vi "UI Main.vi"() -> ()   [LabVIEW 2020]
uses:
  controls/Control Configuration.ctl
  controls/UI Data.ctl
  controls/All FPGA Configuration Values.ctl
  controls/FPGA State.ctl
  controls/Raw Values.ctl
  Globals/Global - All UI Loop Stop.vi
  Globals/Global - UI Stream and Variable Connections.vi
  Globals/Global - Configuration Options.vi
  support/User Event - Stop/User Event - Stop.lvlib
  support/Message Queue/Message Queue.lvlib
panel:
  in  "Switch to Safe State":bool
  in  "Exit":bool
  out "System Status":string
  out "Current FPGA Control Mode":u16(ring) items=["Safe State", "Manual", "Control (PID)"]
  in  "Settings Tab":T1(tab)
  in  "Channel 3 Setpoint":fxp<+/-,16,5>
  in  "Channel 2 Setpoint":fxp<+/-,16,5>
  in  "Channel 1 Setpoint":fxp<+/-,16,5>
  in  "Channel 0 Setpoint":fxp<+/-,16,5>
  in  "Update Control Configuration":bool
  in  "Control Configurations":T2[](array[typedef])
  in  "Run Control":bool
  in  "Stop Control":bool
  in  "Channel 3 Manual Value":fxp<+/-,16,5>
  in  "Channel 2 Manual Value":fxp<+/-,16,5>
  in  "Channel 1 Manual Value":fxp<+/-,16,5>
  in  "Channel 0 Manual Value":fxp<+/-,16,5>
  in  "Run Manual":bool
  in  "Stop Manual":bool
  out "Input Values":T3(graph)
  out "Output Values":T3(graph)
  out "Actual Loop Period (ticks)":u32
  out "Largest Contiguous Memory (bytes)":dbl(graph)
  out "CPU Usage (%)":dbl(graph)
  out "Connected?":bool
  in  "Connect to Controller":bool
  in  "Controller Address":string
  # "LabVIEW FPGA Control on CompactRIO"
  # "Connection Settings"
  # "Element 0 - Chan 0\nElement 1 - Chan 1\nElement 2 - Chan 2\nElement 3 - Chan 3"
  # "Setpoint changes are sent to the target automatically."
  # "Control Configuration changes are sent to the target when you click \"Update Control Configurations\"."
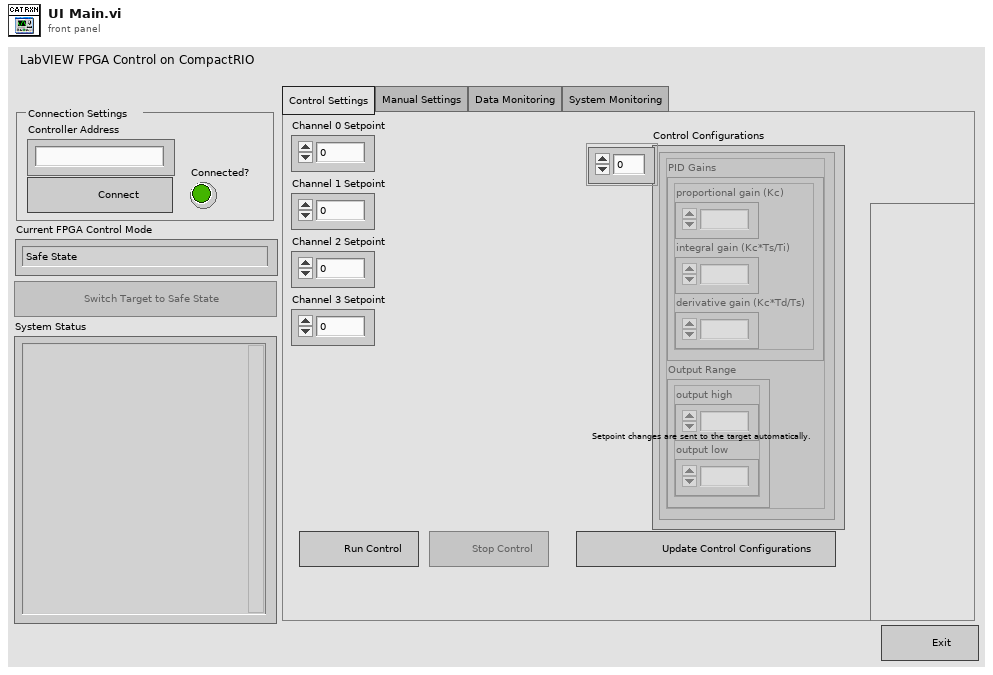
[diagram p1: front panel]
types:
  T1 = enum32{"Control Settings", "Manual Settings", "Data Monitoring", "System Monitoring"}
  T2 = typedef "Control Configuration.ctl" = cluster{"PID Gains":cluster{"proportional gain (Kc)":fxp<+/-,16,8>, "integral gain (Kc*Ts/Ti)":fxp<+/-,16,8>, "derivative gain (Kc*Td/Ts)":fxp<+/-,16,8>}, "Output Range":cluster{"output high":fxp<+/-,16,5>, "output low":fxp<+/-,16,5>}}
  T3 = cluster{"Channel 0":dbl, "Channel 1":dbl, "Channel 2":dbl, "Channel 3":dbl}
  T4 = typedef "UI Data.ctl" = cluster{"Switch to Safe State Ref":refnum<vi>, "Run Manual Ref":refnum<vi>, "Stop Manual Ref":refnum<vi>, "Run Control Ref":refnum<vi>, "Stop Control Ref":refnum<vi>, "Update Control Configurations Ref":refnum<vi>, "Ch 0 Setpoint Ref":refnum<vi>, "Ch 1 Setpoint Ref":refnum<vi>, "Ch 2 Setpoint Ref":refnum<vi>, "Ch 3 Setpoint Ref":refnum<vi>, "Ch 0 Manual Ref":refnum<vi>, "Ch 1 Manual Ref":refnum<vi>, "Ch 2 Manual Ref":refnum<vi>, "Ch 3 Manual Ref":refnum<vi>, "Control Configurations Ref":refnum<vi>}
  T5 = typedef "Message Queue.lvlib/All Message Queues.ctl" = cluster{"UI":refnum<queue>}
  T6 = cluster{"Channel 0 Setpoint":fxp<+/-,16,5>, "Channel 1 Setpoint":fxp<+/-,16,5>, "Channel 2 Setpoint":fxp<+/-,16,5>, "Channel 3 Setpoint":fxp<+/-,16,5>}
  T7 = cluster{"Channel 0 Manual Value":fxp<+/-,16,5>, "Channel 1 Manual Value":fxp<+/-,16,5>, "Channel 2 Manual Value":fxp<+/-,16,5>, "Channel 3 Manual Value":fxp<+/-,16,5>}
  T8 = cluster{"Message":string, "Message Data":variant}
  T9 = typedef "All FPGA Configuration Values.ctl" = cluster{"FPGA State":T10, "Manual Values":T11, "Setpoints":T11, "Control Configurations":T2[]}
  T10 = typedef "FPGA State.ctl" = enum16{"Safe State", "Manual", "Control (PID)"}
  T11 = typedef "Raw Values.ctl" = cluster{"Channel 0":fxp<+/-,20,5>, "Channel 1":fxp<+/-,20,5>, "Channel 2":fxp<+/-,20,5>, "Channel 3":fxp<+/-,20,5>}
  T12 = typedef "Variable References.ctl" = cluster{"CPU Usage":refnum<k21>, "Contiguous Memory":refnum<k21>, "Input Values":refnum<k21>, "Output Values":refnum<k21>, "FPGA Mode":refnum<k21>, "Actual Loop Period":refnum<k21>}
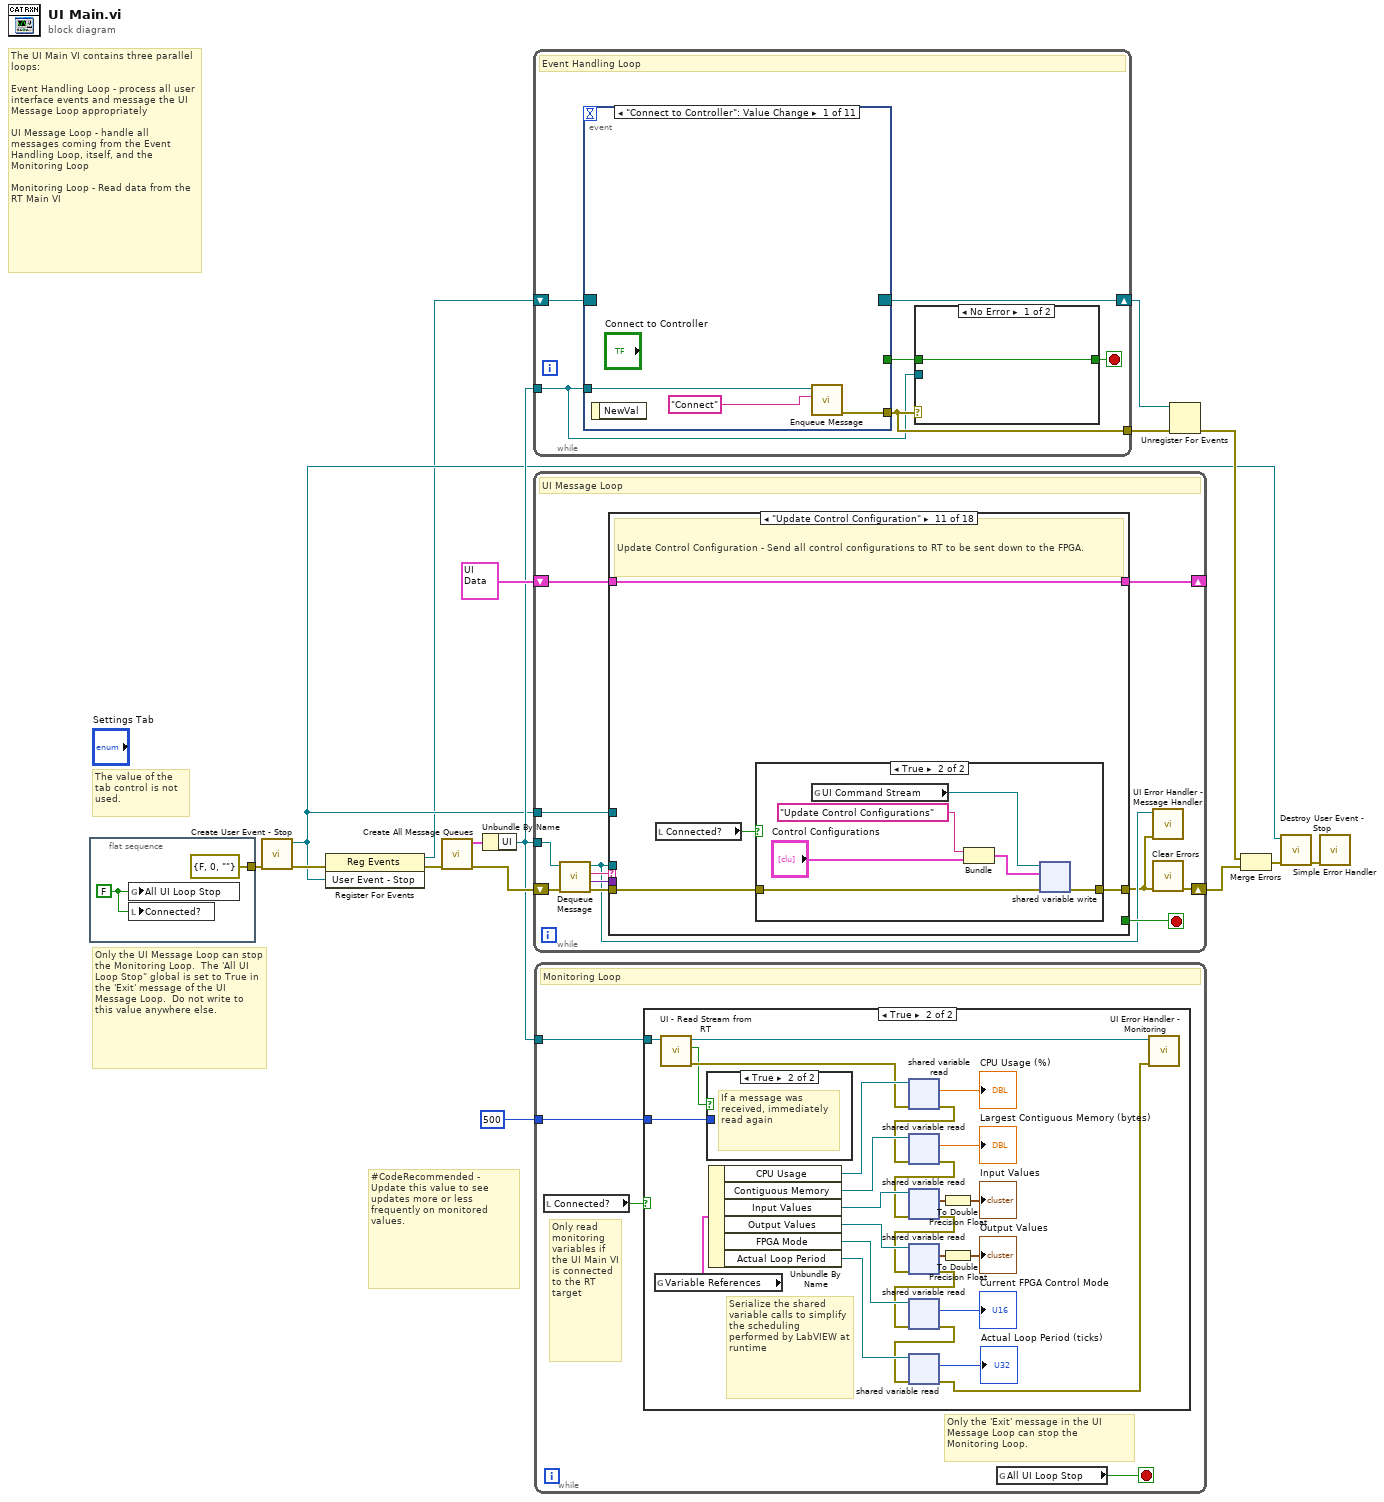
[diagram p0: block diagram]
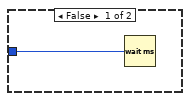
[diagram p2: hidden frame]
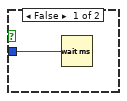
[diagram p3: hidden frame]
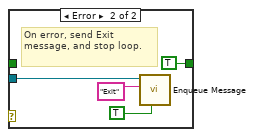
[diagram p4: hidden frame]
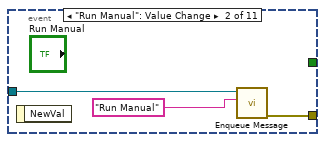
[diagram p5: hidden frame]
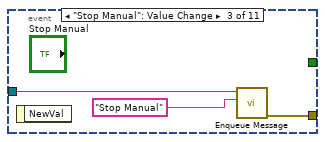
[diagram p6: hidden frame]
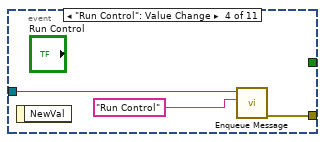
[diagram p7: hidden frame]
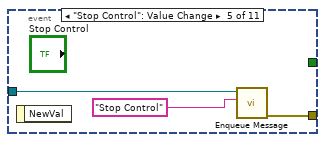
[diagram p8: hidden frame]
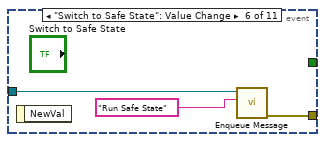
[diagram p9: hidden frame]
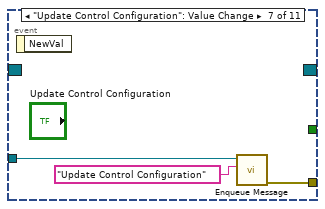
[diagram p10: hidden frame]
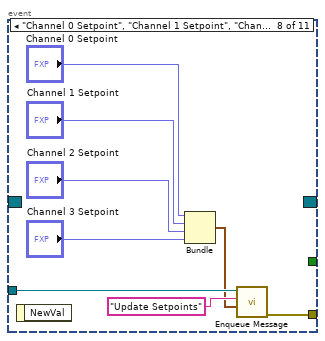
[diagram p11: hidden frame]
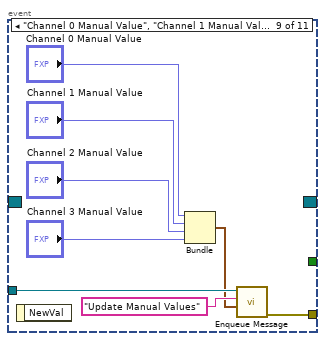
[diagram p12: hidden frame]
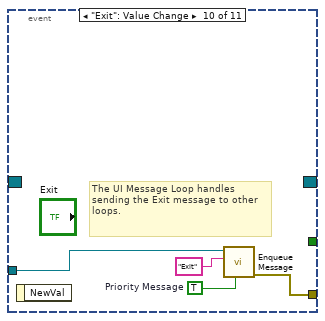
[diagram p13: hidden frame]
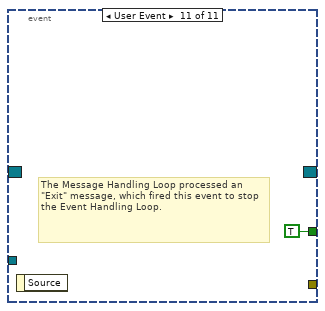
[diagram p14: hidden frame]
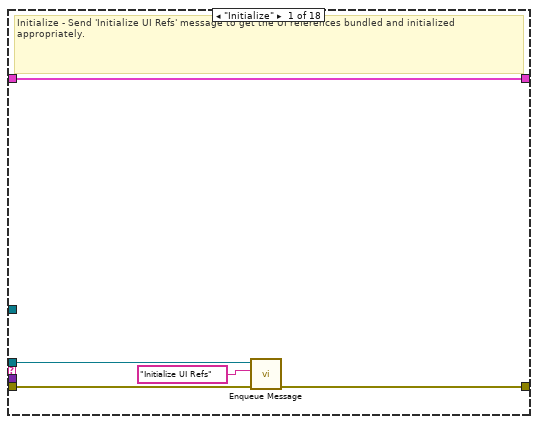
[diagram p15: hidden frame]
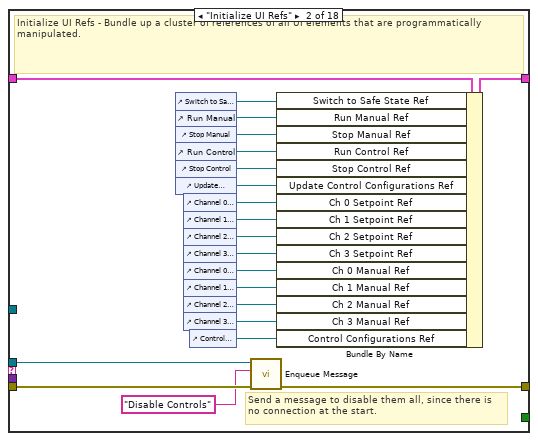
[diagram p16: hidden frame]
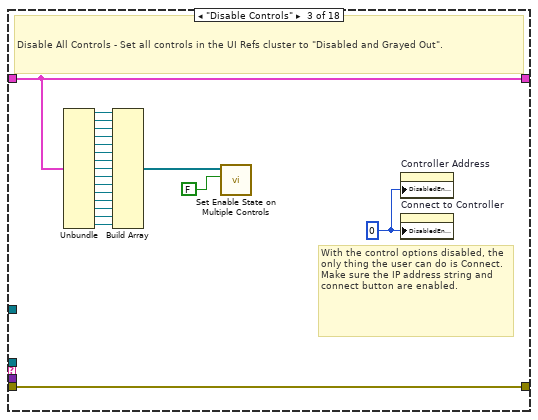
[diagram p17: hidden frame]
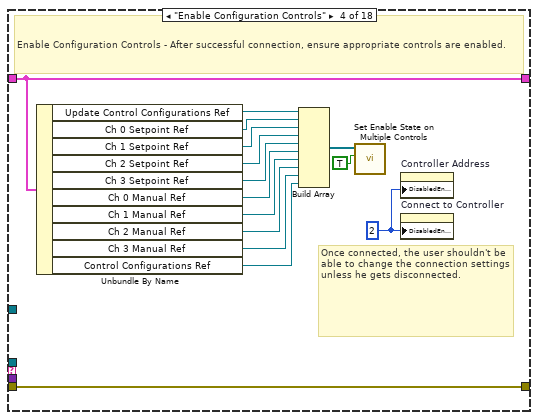
[diagram p18: hidden frame]
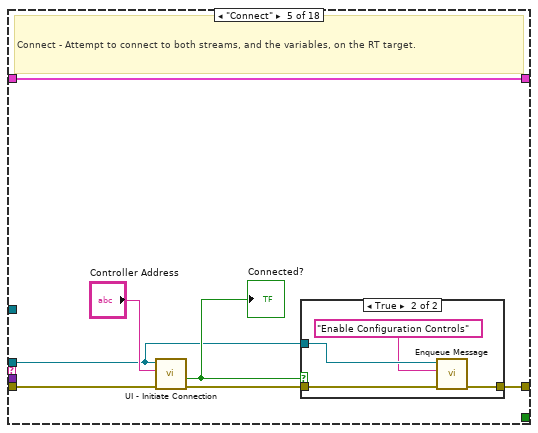
[diagram p19: hidden frame]
diagram:
  # "#CodeRecommended - Update this value to see updates more or less frequently on monitored values."
  # "The UI Main VI contains three parallel loops:\n\nEvent Handling Loop - process all user interface events and message the UI Message Loop appropriately\n\nUI Message Loop - handle all messages coming from the Event Handling Loop, itself, and the Monitoring Loop\n\nMonitoring Loop - Read data from the RT Main VI"
  # "The value of the tab control is not used."
  # "Only the UI Message Loop can stop the Monitoring Loop.  The 'All UI Loop Stop\" global is set to True in the 'Exit' message of the UI Message Loop.  Do not write to this value anywhere else."
  n1 = flat-sequence {
    tunnel: [errorcluster {"status"=FALSE, "code"=0, "source"=""} ("error in (no error)")] -> w6
    frame #0 {
      w17 = FALSE
      n2 = global write "Global - All UI Loop Stop.vi" "All UI Loop Stop"(w17) -> ()
      n3 = local write "Connected?"(w17) -> ()
    }
  }
  n4 = call "Create User Event - Stop.vi"("error in (no error)"=w6) -> ("error out"=w4:errorcluster, "User Event - Stop"=w2:refnum<user-event>)  [unwired: 9 in]
  n5 = register-events(error in=w4, w2) -> (reference out=w1:refnum<event-registration>, error out=w3:errorcluster)  [unwired: 1 in]
  n6 = call "Create All Message Queues.vi"("error in (no error)"=w3) -> ("error out"=w12:errorcluster, "Message Queues out"=w13:T5)  [unwired: 9 in]
  n7 = Unbundle By Name(w13) -> ("UI"=w7:refnum<queue>)
  n8 = while {
    tunnel: w7 -> [w20]
    tunnel: [w22] -> w15
    shift-right: [w19] -> w10
    shift-left: w1 -> [w21]
    stop <- w23 stop-if-true
    # "Event Handling Loop"
    n9 = event shown="[0] \"Connect to Controller\": Value Change" {
      selector: w21 -> [_ _ _ _ _ _ _ _ _ _ _]
      dyn-events: [_ _ _ _ _ _ _ _ _ _ _] -> w19
      timeout: _ -> [_ _ _ _ _ _ _ _ _ _ _]
      tunnel: [_ _ _ _ _ _ _ _ _ _ TRUE ("Discard?")] -> w24
      tunnel: w20 -> [w30 w33 w36 w39 w42 w45 w50 w53 w62 w67 _]
      tunnel: [w32 w35 w38 w41 w44 w47 w49 w52 w61 w70 _] -> w22
      event "Connect to Controller": Value Change {
        n10 = event-data() -> ()  [unwired: 1 in, 1 out]
        n11 = call "Enqueue Message.vi"("Message"="Connect", "Message Queue"=w30) -> ("error out"=w32:errorcluster)  [unwired: 8 in, 1 out]
      }
      event "Run Manual": Value Change {
        n12 = event-data() -> ()  [unwired: 1 in, 1 out]
        n13 = call "Enqueue Message.vi"("Message"="Run Manual", "Message Queue"=w33) -> ("error out"=w35:errorcluster)  [unwired: 8 in, 1 out]
      }
      event "Stop Manual": Value Change {
        n14 = event-data() -> ()  [unwired: 1 in, 1 out]
        n15 = call "Enqueue Message.vi"("Message"="Stop Manual", "Message Queue"=w36) -> ("error out"=w38:errorcluster)  [unwired: 8 in, 1 out]
      }
      event "Run Control": Value Change {
        n16 = event-data() -> ()  [unwired: 1 in, 1 out]
        n17 = call "Enqueue Message.vi"("Message"="Run Control", "Message Queue"=w39) -> ("error out"=w41:errorcluster)  [unwired: 8 in, 1 out]
      }
      event "Stop Control": Value Change {
        n18 = event-data() -> ()  [unwired: 1 in, 1 out]
        n19 = call "Enqueue Message.vi"("Message"="Stop Control", "Message Queue"=w42) -> ("error out"=w44:errorcluster)  [unwired: 8 in, 1 out]
      }
      event "Switch to Safe State": Value Change {
        n20 = event-data() -> ()  [unwired: 1 in, 1 out]
        n21 = call "Enqueue Message.vi"("Message"="Run Safe State", "Message Queue"=w45) -> ("error out"=w47:errorcluster)  [unwired: 8 in, 1 out]
      }
      event "Update Control Configuration": Value Change {
        n22 = event-data() -> ()  [unwired: 1 in, 1 out]
        n23 = call "Enqueue Message.vi"("Message"="Update Control Configuration", "Message Queue"=w50) -> ("error out"=w49:errorcluster)  [unwired: 8 in, 1 out]
      }
      event "Channel 0 Setpoint", "Channel 1 Setpoint", "Channel 2 Setpoint", "Channel 3 Setpoint": Value Change {
        n24 = event-data() -> ()  [unwired: 1 in, 1 out]
        n25 = Bundle("Channel 0 Setpoint"="Channel 0 Setpoint", "Channel 1 Setpoint"="Channel 1 Setpoint", "Channel 2 Setpoint"="Channel 2 Setpoint", "Channel 3 Setpoint"="Channel 3 Setpoint") -> (w51:T6)  [unwired: 1 in]
        n26 = call "Enqueue Message.vi"("Message Data"=w51, "Message"="Update Setpoints", "Message Queue"=w53) -> ("error out"=w52:errorcluster)  [unwired: 7 in, 1 out]
      }
      event "Channel 0 Manual Value", "Channel 1 Manual Value", "Channel 2 Manual Value", "Channel 3 Manual Value": Value Change {
        n27 = event-data() -> ()  [unwired: 1 in, 1 out]
        n28 = Bundle("Channel 0 Manual Value"="Channel 0 Manual Value", "Channel 1 Manual Value"="Channel 1 Manual Value", "Channel 2 Manual Value"="Channel 2 Manual Value", "Channel 3 Manual Value"="Channel 3 Manual Value") -> (w59:T7)  [unwired: 1 in]
        n29 = call "Enqueue Message.vi"("Message Data"=w59, "Message"="Update Manual Values", "Message Queue"=w62) -> ("error out"=w61:errorcluster)  [unwired: 7 in, 1 out]
      }
      event "Exit": Value Change {
        w68 = TRUE  # Priority Message
        # "The UI Message Loop handles sending the Exit message to other loops."
        n30 = event-data() -> ()  [unwired: 1 in, 1 out]
        n31 = call "Enqueue Message.vi"("Priority Message? (F)"=w68, "Message"="Exit", "Message Queue"=w67) -> ("error out"=w70:errorcluster)  [unwired: 7 in, 1 out]
      }
      event User Event {
        # "The Message Handling Loop processed an \"Exit\" message, which fired this event to stop the Event Handling Loop."
        n32 = event-data() -> ()  [unwired: 1 in, 1 out]
      }
    }
    n33 = case shown="No Error" w22 {
      tunnel: [w25 TRUE ("Discard?")] -> w23
      tunnel: w24 -> [w25 _]
      tunnel: w20 -> [_ w26]
      frame No Error {
      }
      frame Error {
        # "On error, send Exit message, and stop loop."
        n34 = call "Enqueue Message.vi"("Priority Message? (F)"=TRUE ("Discard?"), "Message"="Exit", "Message Queue"=w26) -> ()  [unwired: 7 in, 2 out]
      }
    }
  }
  n35 = while {
    tunnel: w7 -> [w77]
    tunnel: w2 -> [w82]
    shift-right: [w72] -> w16
    shift-left: w12 -> [w81]
    shift-right: [w75] -> _
    shift-left: T4 {"Switch to Safe State Ref"=refnum, "Run Manual Ref"=refnum, "Stop Manual Ref"=refnum, "Run Control Ref"=refnum, "Stop Control Ref"=refnum, "Update Control Configurations Ref"=refnum, "Ch 0 Setpoint Ref"=refnum, "Ch 1 Setpoint Ref"=refnum, "Ch 2 Setpoint Ref"=refnum, "Ch 3 Setpoint Ref"=refnum, "Ch 0 Manual Ref"=refnum, "Ch 1 Manual Ref"=refnum, "Ch 2 Manual Ref"=refnum, "Ch 3 Manual Ref"=refnum, "Control Configurations Ref"=refnum} ("Measurement UI Controls") -> [w76]
    stop <- w83 stop-if-true
    # "UI Message Loop"
    n36 = call "Dequeue Message.vi"("error in (no error)"=w81, "Message Queue"=w77) -> ("error out"=w80:errorcluster, "Message Data"=w78:variant, "Message"=w79:string, "dup Message Queue"=w74:refnum<queue>)  [unwired: 6 in]
    n37 = case "Message Cases" shown="\"Update Control Configuration\"" w79 {
      selector: w79 -> [_ _ _ _ _ _ _ _ _ w206 _ w238 _ w288 _ _ _ w349]
      tunnel: w74 -> [w85 w90 _ _ w146 _ w164 _ w178 w207 _ _ _ w292 _ w334 _ _]
      tunnel: w80 -> [w87 w109 w129 w130 w151 w162 w166 w171 w202 w209 w227 w239 w259 w302 w323 w339 w344 _]
      tunnel: [w86 w91 w129 w130 w145 w162 w165 w170 w181 w208 w226 w240 w258 w303 w321 w340 w343 w347] -> w73
      tunnel: [_ _ _ _ _ _ _ _ _ _ _ _ _ _ _ TRUE _ _] -> w83
      tunnel: w78 -> [_ _ _ _ _ _ _ _ w200 _ _ w237 w257 w300 w320 _ _ _]
      tunnel: w82 -> [_ _ _ _ _ _ _ _ _ _ _ _ _ _ _ w338 _ _]
      tunnel: w76 -> [w88 w108 w128 w141 w150 w161 w168 w172 w197 w210 w228 w241 w256 w304 w322 w336 w342 w345]
      tunnel: [w88 w107 w128 w141 w150 w161 w168 w172 w197 w210 w228 w241 w256 w304 w322 w336 w342 w345] -> w75
      frame "Initialize" {
        # "Initialize - Send 'Initialize UI Refs' message to get the UI references bundled and initialized appropriately."
        n38 = call "Enqueue Message.vi"("error in (no error)"=w87, "Message"="Initialize UI Refs", "Message Queue"=w85) -> ("error out"=w86:errorcluster)  [unwired: 7 in, 1 out]
      }
      frame "Initialize UI Refs" {
        # "Send a message to disable them all, since there is no connection at the start."
        # "Initialize UI Refs - Bundle up a cluster of references of all UI elements that are programmatically manipulated."
        n39 = control-ref of="Switch to Safe State"() -> (w106:refnum<vi>)
        n40 = control-ref of="Run Manual"() -> (w105:refnum<vi>)
        n41 = control-ref of="Stop Manual"() -> (w104:refnum<vi>)
        n42 = control-ref of="Run Control"() -> (w103:refnum<vi>)
        n43 = control-ref of="Stop Control"() -> (w102:refnum<vi>)
        n44 = control-ref of="Update Control Configuration"() -> (w101:refnum<vi>)
        n45 = control-ref of="Channel 0 Setpoint"() -> (w100:refnum<vi>)
        n46 = control-ref of="Channel 1 Setpoint"() -> (w99:refnum<vi>)
        n47 = control-ref of="Channel 2 Setpoint"() -> (w98:refnum<vi>)
        n48 = control-ref of="Channel 3 Setpoint"() -> (w97:refnum<vi>)
        n49 = control-ref of="Channel 0 Manual Value"() -> (w96:refnum<vi>)
        n50 = control-ref of="Channel 1 Manual Value"() -> (w95:refnum<vi>)
        n51 = control-ref of="Channel 2 Manual Value"() -> (w94:refnum<vi>)
        n52 = control-ref of="Channel 3 Manual Value"() -> (w93:refnum<vi>)
        n53 = control-ref of="Control Configurations"() -> (w92:refnum<vi>)
        n54 = call "Enqueue Message.vi"("error in (no error)"=w109, "Message"="Disable Controls", "Message Queue"=w90) -> ("error out"=w91:errorcluster)  [unwired: 7 in, 1 out]
        n55 = Bundle By Name(cluster=w108, "Switch to Safe State Ref"=w106, "Run Manual Ref"=w105, "Stop Manual Ref"=w104, "Run Control Ref"=w103, "Stop Control Ref"=w102, "Update Control Configurations Ref"=w101, "Ch 0 Setpoint Ref"=w100, "Ch 1 Setpoint Ref"=w99, "Ch 2 Setpoint Ref"=w98, "Ch 3 Setpoint Ref"=w97, "Ch 0 Manual Ref"=w96, "Ch 1 Manual Ref"=w95, "Ch 2 Manual Ref"=w94, "Ch 3 Manual Ref"=w93, "Control Configurations Ref"=w92) -> (w107:T4)
      }
      frame "Disable Controls" {
        w110 = 0
        # "With the control options disabled, the only thing the user can do is Connect. Make sure the IP address string and connect button are enabled."
        # "Disable All Controls - Set all controls in the UI Refs cluster to \"Disabled and Grayed Out\"."
        n56 = Unbundle(w128) -> ("Switch to Safe State Ref"=w127:refnum<vi>, "Run Manual Ref"=w126:refnum<vi>, "Stop Manual Ref"=w125:refnum<vi>, "Run Control Ref"=w124:refnum<vi>, "Stop Control Ref"=w123:refnum<vi>, "Update Control Configurations Ref"=w122:refnum<vi>, "Ch 0 Setpoint Ref"=w121:refnum<vi>, "Ch 1 Setpoint Ref"=w120:refnum<vi>, "Ch 2 Setpoint Ref"=w119:refnum<vi>, "Ch 3 Setpoint Ref"=w118:refnum<vi>, "Ch 0 Manual Ref"=w117:refnum<vi>, "Ch 1 Manual Ref"=w116:refnum<vi>, "Ch 2 Manual Ref"=w115:refnum<vi>, "Ch 3 Manual Ref"=w114:refnum<vi>, "Control Configurations Ref"=w113:refnum<vi>)
        n57 = Build Array(w127, w126, w125, w124, w123, w122, w121, w120, w119, w118, w117, w116, w115, w114, w113) -> (w112:refnum<vi>[])
        n58 = call "Set Enable State on Multiple Controls.vi"("Enable?"=FALSE, "Controls"=w112) -> ()  [unwired: 10 in]
        n59 = property on="Controller Address" class="Str"("DisabledEnum"=w110) -> ()  [unwired: 2 in, 2 out]
        n60 = property on="Connect to Controller" class="Bool"("DisabledEnum"=w110) -> ()  [unwired: 2 in, 2 out]
      }
      frame "Enable Configuration Controls" {
        w142 = 2
        # "Once connected, the user shouldn't be able to change the connection settings unless he gets disconnected."
        # "Enable Configuration Controls - After successful connection, ensure appropriate controls are enabled."
        n61 = Unbundle By Name(w141) -> ("Update Control Configurations Ref"=w140:refnum<vi>, "Ch 0 Setpoint Ref"=w139:refnum<vi>, "Ch 1 Setpoint Ref"=w138:refnum<vi>, "Ch 2 Setpoint Ref"=w137:refnum<vi>, "Ch 3 Setpoint Ref"=w136:refnum<vi>, "Ch 0 Manual Ref"=w135:refnum<vi>, "Ch 1 Manual Ref"=w134:refnum<vi>, "Ch 2 Manual Ref"=w133:refnum<vi>, "Ch 3 Manual Ref"=w132:refnum<vi>, "Control Configurations Ref"=w131:refnum<vi>)
        n62 = Build Array(w140, w139, w138, w137, w136, w135, w134, w133, w132, w131) -> (w144:refnum<vi>[])
        n63 = call "Set Enable State on Multiple Controls.vi"("Enable?"=TRUE, "Controls"=w144) -> ()  [unwired: 10 in]
        n64 = property on="Controller Address" class="Str"("DisabledEnum"=w142) -> ()  [unwired: 2 in, 2 out]
        n65 = property on="Connect to Controller" class="Bool"("DisabledEnum"=w142) -> ()  [unwired: 2 in, 2 out]
      }
      frame "Connect" {
        # "Connect - Attempt to connect to both streams, and the variables, on the RT target."
        n66 = call "UI - Initiate Connection.vi"("error in (no error)"=w151, "Controller Address"="Controller Address", "Message Queue"=w146) -> ("error out"=w148:errorcluster, "Connected?"=w147:bool)  [unwired: 7 in]
        "Connected?" <- w147
        n67 = case shown="True" w147 {
          tunnel: w148 -> [w152 w156]
          tunnel: w146 -> [_ w155]
          tunnel: [w152 w154] -> w145
          frame False {
          }
          frame True {
            n68 = call "Enqueue Message.vi"("error in (no error)"=w156, "Message"="Enable Configuration Controls", "Message Queue"=w155) -> ("error out"=w154:errorcluster)  [unwired: 7 in, 1 out]
          }
        }
      }
      frame "Close Connections" {
        # "Close Connections - Close the connections shared with the Monitoring Loop."
        n69 = global read "Global - UI Stream and Variable Connections.vi" "UI Command Stream"() -> (w160:refnum<k21>)
        n70 = global read "Global - UI Stream and Variable Connections.vi" "RT Message Stream"() -> (w159:refnum<k21>)
        n71 = global read "Global - UI Stream and Variable Connections.vi" "Variable References"() -> (w158:T12)
        n72 = local write "Connected?"(FALSE ("Connected?")) -> ()
        n73 = Destroy Stream Endpoint(11:w160) -> ()  [unwired: 1 in, 1 out]
        n74 = Destroy Stream Endpoint(11:w159) -> ()  [unwired: 1 in, 1 out]
        n75 = call "Close Variable Connections.vi"("Variable References"=w158) -> ()  [unwired: 11 in]
      }
      frame "Disconnect UI" {
        # "Disconnect UI - Something has gone wrong with the connection. Reinitialize the UI to its disconnected state."
        n76 = local write "Connected?"(FALSE ("Connected?")) -> ()
        n77 = call "Enqueue Message.vi"("error in (no error)"=w166, "Message"="Disable Controls", "Message Queue"=w164) -> ("error out"=w165:errorcluster)  [unwired: 7 in, 1 out]
      }
      frame "Get Settings from FPGA" {
        # "Get Settings from FPGA - Send a command to the RT to retrieve all current FPGA Main VI parameter values and send them back to the UI."
        n78 = local read "Connected?"() -> (w169:bool)
        n79 = case shown="True" w169 {
          tunnel: w171 -> [w173 w177]
          tunnel: [w173 w176] -> w170
          frame False {
            # "Don't bother trying to send a message to the RT system if UI Main VI isn't even connected"
          }
          frame True {
            n80 = global read "Global - UI Stream and Variable Connections.vi" "UI Command Stream"() -> (w174:refnum<k21>)
            n81 = shared-variable-write(w174, w177, T8 {"Message"="Send FPGA Configuration to UI", "Message Data"=variant} ("data in")) -> (w176:errorcluster)  [unwired: 1 in, 2 out]
          }
        }
      }
      frame "Initial UI Values" {
        # "Set values of all manual and setpoint controls via reference."
        # "Initial UI Values - These are the current values of the FPGA Main VI's R/W controls. They are used to initialize the panel of UI Main VI upon successful connection to the RT target."
        n82 = Variant To Data(error in=w202, type=T9 {"FPGA State"=enum."Safe State", "Manual Values"={"Channel 0"=0.0, "Channel 1"=0.0, "Channel 2"=0.0, "Channel 3"=0.0}, "Setpoints"={"Channel 0"=0.0, "Channel 1"=0.0, "Channel 2"=0.0, "Channel 3"=0.0}, "Control Configurations"=[]} ("All FPGA Configuration Values"), Variant=w200) -> (data=w198:T9, error out=w201:errorcluster)
        n83 = Unbundle By Name(w197) -> ("Ch 0 Setpoint Ref"=w192:refnum<vi>, "Ch 1 Setpoint Ref"=w191:refnum<vi>, "Ch 2 Setpoint Ref"=w190:refnum<vi>, "Ch 3 Setpoint Ref"=w189:refnum<vi>, "Ch 0 Manual Ref"=w188:refnum<vi>, "Ch 1 Manual Ref"=w187:refnum<vi>, "Ch 2 Manual Ref"=w186:refnum<vi>, "Ch 3 Manual Ref"=w185:refnum<vi>)
        n84 = Unbundle By Name(w198) -> ("Setpoints"=w196:T11, "Manual Values"=w195:T11, "Control Configurations"=w182:T2[], "FPGA State"=w179:T10)
        n85 = Build Array(w192, w191, w190, w189, w188, w187, w186, w185) -> (w184:refnum<vi>[])
        n86 = Cluster To Array(cluster=w196) -> (array=w194:fxp<+/-,20,5>[])
        n87 = Cluster To Array(cluster=w195) -> (array=w193:fxp<+/-,20,5>[])
        n88 = local write "Current FPGA Control Mode"(w179) -> ()
        n89 = Build Array (concatenate)(w194, w193) -> (w183:fxp<+/-,20,5>[])
        n90 = local write "Control Configurations"(w182) -> ()
        n91 = for {
          tunnel: w184 -> [w204] mode=indexing
          tunnel: w183 -> [w203] mode=indexing
          n92 = property class="DigNum"(reference=w204, "Value"=w203) -> ()  [unwired: 1 in, 2 out]
        }
        n93 = call "Enqueue Message.vi"("error in (no error)"=w201, "Message Data"=w179, "Message"="Update Display Mode", "Message Queue"=w178) -> ("error out"=w181:errorcluster)  [unwired: 6 in, 1 out]
      }
      frame "Run Control", "Run Manual", "Run Safe State", "Stop Control", "Stop Manual" {
        # "Run/Stop buttons - Send a command to switch the FPGA into the appropriate state. Send a message to update this UI to reflect the new state."
        n94 = local read "Connected?"() -> (w205:bool)
        n95 = case shown="True" w205 {
          tunnel: w209 -> [w211 w221]
          tunnel: [w211 w217] -> w208
          tunnel: w207 -> [_ w216]
          tunnel: w206 -> [_ w215]
          frame False {
            # "Don't bother trying to send a message to the RT system if UI Main VI isn't even connected"
          }
          frame True {
            # "Run Manual and Run Control switch into their respective states. Anything else switches to Safe State."
            n96 = case shown="\"Safe State\", \"Stop Control\", \"Stop Manual\", Default" w215 {
              tunnel: [FPGA_State."Safe State" ("FPGA State") FPGA_State."Control (PID)" ("FPGA State") FPGA_State."Manual" ("FPGA State")] -> w212
              frame "Safe State", "Stop Control", "Stop Manual", Default {
              }
              frame "Run Control" {
              }
              frame "Run Manual" {
              }
            }
            n97 = global read "Global - UI Stream and Variable Connections.vi" "UI Command Stream"() -> (w213:refnum<k21>)
            n98 = Bundle("Update FPGA State", "FPGA State"=w212) -> (w218:cluster{string, "FPGA State":T10})  [unwired: 1 in]
            n99 = shared-variable-write(w213, w221, w218) -> (w220:errorcluster)  [unwired: 1 in, 2 out]
            n100 = call "Enqueue Message.vi"("error in (no error)"=w220, "Message Data"=w212, "Message"="Update Display Mode", "Message Queue"=w216) -> ("error out"=w217:errorcluster)  [unwired: 6 in, 1 out]
          }
        }
      }
      frame "Update Control Configuration" {
        # "Update Control Configuration - Send all control configurations to RT to be sent down to the FPGA."
        n101 = local read "Connected?"() -> (w225:bool)
        n102 = case shown="True" w225 {
          tunnel: w227 -> [w229 w235]
          tunnel: [w229 w234] -> w226
          frame False {
            # "Don't bother trying to send a message to the RT system if UI Main VI isn't even connected"
          }
          frame True {
            n103 = global read "Global - UI Stream and Variable Connections.vi" "UI Command Stream"() -> (w230:refnum<k21>)
            n104 = Bundle("Update Control Configurations", "Control Configurations"="Control Configurations") -> (w232:cluster{string, "Control Configurations":T2[]})  [unwired: 1 in]
            n105 = shared-variable-write(w230, w235, w232) -> (w234:errorcluster)  [unwired: 1 in, 2 out]
          }
        }
      }
      frame "Update Manual Values", "Update Setpoints" {
        # "Update Manual Values/Setpoints - Send all manual values/setpoints to RT to be sent down to the FPGA."
        n106 = local read "Connected?"() -> (w236:bool)
        n107 = case shown="True" w236 {
          tunnel: [w242 w248] -> w240
          tunnel: w239 -> [w242 w246]
          tunnel: w238 -> [_ w245]
          tunnel: w237 -> [_ w244]
          frame False {
            # "Don't bother trying to send a message to the RT system if UI Main VI isn't even connected"
          }
          frame True {
            n108 = global read "Global - UI Stream and Variable Connections.vi" "UI Command Stream"() -> (w243:refnum<k21>)
            n109 = Bundle(w245, "Message Data"=w244) -> (w247:cluster{string, "Message Data":variant})  [unwired: 1 in]
            n110 = shared-variable-write(w243, w246, w247) -> (w248:errorcluster)  [unwired: 1 in, 2 out]
          }
        }
      }
      frame "Update Display Mode" {
        # "Update Display Mode - Enable/Disable Controls appropriately for the new display mode."
        n111 = Variant To Data(error in=w259, type=FPGA_State."Safe State" ("FPGA State"), Variant=w257) -> (data=w255:T10, error out=w258:errorcluster)
        n112 = Unbundle By Name(w256) -> ("Switch to Safe State Ref"=w254:refnum<vi>, "Run Manual Ref"=w253:refnum<vi>, "Stop Manual Ref"=w252:refnum<vi>, "Run Control Ref"=w251:refnum<vi>, "Stop Control Ref"=w250:refnum<vi>)
        n113 = case shown="\"Manual\"" w255 {
          tunnel: w254 -> [w264 w273 w280]
          tunnel: w253 -> [w260 w272 w282]
          tunnel: w252 -> [w263 w271 w279]
          tunnel: w251 -> [w262 w269 w281]
          tunnel: w250 -> [w261 w270 w278]
          frame "Control (PID)" {
            n114 = Build Array "Controls to Enable"(w264, w261, w260) -> (w268:refnum<vi>[])
            n115 = Build Array "Controls to Disable"(w263, w262) -> (w266:refnum<vi>[])
            n116 = call "Set Enable State on Multiple Controls.vi"("Enable?"=FALSE, "Controls"=w266) -> ()  [unwired: 10 in]
            n117 = call "Set Enable State on Multiple Controls.vi"("Enable?"=TRUE, "Controls"=w268) -> ()  [unwired: 10 in]
          }
          frame "Manual" {
            n118 = Build Array "Controls to Enable"(w273, w271, w269) -> (w277:refnum<vi>[])
            n119 = Build Array "Controls to Disable"(w272, w270) -> (w275:refnum<vi>[])
            n120 = call "Set Enable State on Multiple Controls.vi"("Enable?"=FALSE, "Controls"=w275) -> ()  [unwired: 10 in]
            n121 = call "Set Enable State on Multiple Controls.vi"("Enable?"=TRUE, "Controls"=w277) -> ()  [unwired: 10 in]
          }
          frame "Safe State" {
            # "This frame runs when FPGA is in Safe State. Only enable the two run buttons."
            n122 = Build Array "Controls to Enable"(w282, w281) -> (w286:refnum<vi>[])
            n123 = Build Array "Controls to Disable"(w280, w279, w278) -> (w284:refnum<vi>[])
            n124 = call "Set Enable State on Multiple Controls.vi"("Enable?"=FALSE, "Controls"=w284) -> ()  [unwired: 10 in]
            n125 = call "Set Enable State on Multiple Controls.vi"("Enable?"=TRUE, "Controls"=w286) -> ()  [unwired: 10 in]
          }
        }
      }
      frame "Critical Error", "Log-Only Error", "Non-Critical Error", "RT Error" {
        # "Error - Display message in status indicator on panel.  If it's a critical error, shut down this VI with an 'Exit' message."
        n126 = case shown="Default" w288 {
          selector: w288 -> [_ w306]
          tunnel: ["UI Error" w306] -> w287
          frame Default {
          }
          frame "RT Error" {
          }
        }
        n127 = Variant To Data(error in=w302, type=errorcluster {"status"=FALSE, "code"=0, "source"=""} ("error constant"), Variant=w300) -> (data=w295:errorcluster, error out=w301:errorcluster)
        n128 = Unbundle By Name(w295) -> ("code"=w294:i32, "source"=w298:string)
        n129 = Format Date/Time String() -> (date/time string=w297:string)  [unwired: 3 in]
        n130 = Format Into String(format string="\n%s: %s %d - %s", w297, w287, w294, w298) -> (resulting string=w289:string)  [unwired: 2 in, 1 out]
        n131 = call "Enqueue Message.vi"("error in (no error)"=w301, "Message Data"=w289, "Message"="Update System Status", "Message Queue"=w292) -> ("error out"=w293:errorcluster, "dup Message Queue"=w291:refnum<queue>)  [unwired: 6 in]
        n132 = case shown="Default" w288 {
          tunnel: w293 -> [w307 w311]
          tunnel: w291 -> [_ w309]
          tunnel: [w307 w310] -> w303
          frame Default {
          }
          frame "Critical Error" {
            n133 = call "Enqueue Message.vi"("error in (no error)"=w311, "Message"="Exit", "Message Queue"=w309) -> ("error out"=w310:errorcluster)  [unwired: 7 in, 1 out]
          }
        }
      }
      frame "Update System Status" {
        # "#CodeRecommended - The code below ensures that the System Status string value does not become too large.  It uses the same maximum size as the RT error log to determine whether or not to remove the last half of the log string. Change this logic if you wish to maintain more/less of the information in the System Status string."
        # "Update System Status - Add a new string to the beginning of the System Status string on the UI."
        n134 = Variant To Data(error in=w323, type="", Variant=w320) -> (data=w317:string, error out=w321:errorcluster)
        n135 = local read "System Status"() -> (w315:string)
        n136 = global read "Global - Configuration Options.vi" "Error Log Max Size (bytes)"() -> (w313:i64)
        n137 = String Length(string=w315) -> (length=w316:i32)
        n138 = Greater?(x=w316, y=w313) -> (0:w314:bool)
        n139 = case shown="True" w314 {
          tunnel: w315 -> [w324 w328]
          tunnel: w313 -> [_ w327]
          tunnel: [w324 w329] -> w312
          frame False {
          }
          frame True {
            n140 = Divide(x=w327, y=i64 2) -> (x/y=w326:dbl)
            n141 = String Subset(string=w328, length (rest)=w326) -> (substring=w329:string)  [unwired: 1 in]
          }
        }
        n142 = Concatenate Strings(w317, w312) -> (→"System Status":string)
      }
      frame "Exit" {
        # "Close all connections"
        # "Stop Monitoring Loop"
        # "Stop Event Handling Loop"
        # "Release the UI Message queue reference"
        # "Stop UI Message Loop"
        # "Exit - Fire the User Event to stop the Event Handling Loop, and toggle the local variable to stop the Monitoring Loop.  This message alone causes all three loops to stop."
        n143 = global write "Global - All UI Loop Stop.vi" "All UI Loop Stop"(TRUE ("Stop Monitoring Loop")) -> ()
        n144 = call "Fire User Event - Stop.vi"("User Event - Stop"=w338) -> ("error out"=w337:errorcluster)  [unwired: 10 in]
        n145 = Release Queue(queue=w334, error in (no error)=w339) -> (error out=w335:errorcluster)  [unwired: 1 in, 2 out]
        n146 = global read "Global - UI Stream and Variable Connections.vi" "UI Command Stream"() -> (w332:refnum<k21>)
        n147 = global read "Global - UI Stream and Variable Connections.vi" "RT Message Stream"() -> (w331:refnum<k21>)
        n148 = global read "Global - UI Stream and Variable Connections.vi" "Variable References"() -> (w330:T12)
        n149 = Destroy Stream Endpoint(11:w332) -> ()  [unwired: 1 in, 1 out]
        n150 = Destroy Stream Endpoint(11:w331) -> ()  [unwired: 1 in, 1 out]
        n151 = call "Close Variable Connections.vi"("Variable References"=w330) -> ()  [unwired: 11 in]
        n152 = Merge Errors(w337, w335) -> (w340:errorcluster)
      }
      frame "---Copy This Frame---" {
        # "Duplicate this frame when creating new messages.  Change this comment in the duplicated frame to describe this message."
        n153 = Merge Errors(w344) -> (w343:errorcluster)
      }
      frame Default {
        # "'Default' case only runs if there is a message that isn't defined in any of the other cases.  Output a programming error."
        n154 = Format Into String(format string="The invalid message string \"%s\" was received in the Message Handling Loop." ("Invalid Message Loop Message"), w349) -> (resulting string=w346:string)  [unwired: 2 in, 1 out]
        n155 = call <vilib>:"Error Cluster From Error Code.vi"("error message (\"\")"=w346, "error code (0)"=1) -> ("error out"=w347:errorcluster)  [unwired: 7 in]
      }
    }
    n156 = call "UI Error Handler - Message Handler.vi"("error in (no error)"=w73, "Message Queue"=w74) -> ()  [unwired: 9 in, 1 out]
    n157 = call <vilib>:"Clear Errors.vi"("error in (no error)"=w73) -> ("error out"=w72:errorcluster)  [unwired: 5 in, 1 out]
  }
  n158 = while {
    tunnel: w7 -> [w353]
    tunnel: u32 500 ("milliseconds to wait") -> [w351]
    stop <- w354 stop-if-true
    # "Only read monitoring variables if the UI Main VI is connected to the RT target"
    # "Only the 'Exit' message in the UI Message Loop can stop the Monitoring Loop."
    # "Monitoring Loop"
    n159 = local read "Connected?"() -> (w352:bool)
    n160 = case shown="True" w352 {
      tunnel: w353 -> [_ w361]
      tunnel: w351 -> [w355 w356]
      frame False {
        n161 = Wait (ms)(milliseconds to wait=w355) -> ()  [unwired: 1 out]
      }
      frame True {
        # "Serialize the shared variable calls to simplify the scheduling performed by LabVIEW at runtime"
        n162 = global read "Global - UI Stream and Variable Connections.vi" "Variable References"() -> (w359:T12)
        n163 = call "UI - Read Stream from RT.vi"("Message Queue"=w361) -> ("error out"=w367:errorcluster, "Message Received?"=w357:bool, "dup Message Queue"=w360:refnum<queue>)  [unwired: 8 in]
        n164 = case shown="True" w357 {
          tunnel: w356 -> [w382 _]
          frame False {
            n165 = Wait (ms)(milliseconds to wait=w382) -> ()  [unwired: 1 out]
          }
          frame True {
            # "If a message was received, immediately read again"
          }
        }
        n166 = Unbundle By Name(w359) -> ("CPU Usage"=w374:refnum<k21>, "Contiguous Memory"=w373:refnum<k21>, "Input Values"=w372:refnum<k21>, "Output Values"=w371:refnum<k21>, "FPGA Mode"=w370:refnum<k21>, "Actual Loop Period"=w369:refnum<k21>)
        n167 = shared-variable-read(w374, w367) -> (w366:errorcluster, →"CPU Usage (%)":dbl)  [unwired: 2 out]
        n168 = shared-variable-read(w373, w366) -> (w365:errorcluster, →"Largest Contiguous Memory (bytes)":dbl)  [unwired: 2 out]
        n169 = shared-variable-read(w372, w365) -> (w364:errorcluster, w377:T11)  [unwired: 2 out]
        n170 = shared-variable-read(w371, w364) -> (w363:errorcluster, w376:T11)  [unwired: 2 out]
        n171 = shared-variable-read(w370, w363) -> (w362:errorcluster, →"Current FPGA Control Mode":T10)  [unwired: 2 out]
        n172 = shared-variable-read(w369, w362) -> (w368:errorcluster, →"Actual Loop Period (ticks)":u32)  [unwired: 2 out]
        n173 = To Double Precision Float(number=w377) -> (double precision float=→"Input Values":T3)
        n174 = To Double Precision Float(number=w376) -> (double precision float=→"Output Values":T3)
        n175 = call "UI Error Handler - Monitoring.vi"("error in (no error)"=w368, "Message Queue"=w360) -> ()  [unwired: 9 in, 1 out]
      }
    }
    n176 = global read "Global - All UI Loop Stop.vi" "All UI Loop Stop"() -> (w354:bool)
  }
  n177 = Unregister For Events(event registration refnum=w10, error in=w15) -> (error out=w11:errorcluster)
  n178 = Merge Errors(w11, w16) -> (w14:errorcluster)
  n179 = call "Destroy User Event - Stop.vi"("error in (no error)"=w14, "User Event - Stop"=w2) -> ("error out"=w8:errorcluster)  [unwired: 9 in]
  n180 = call <vilib>:"Simple Error Handler.vi"("error in (no error)"=w8) -> ()  [unwired: 4 in, 5 out]
